vi "Renishaw-XL80_CancelPreHeat.vi"(8 "error in (no error)":errorcluster, 11 "Renishaw-XL80 in":refnum<class "Renishaw-XL80.lvclass">) -> (0 "error out":errorcluster, 3 "Renishaw-XL80 out":refnum<class "Renishaw-XL80.lvclass">)   [LabVIEW 2024, in "Renishaw-XL80.lvclass"]
doc: "This method will terminate the preheat cycle of the ML10. This method should be used with caution, since shortening the preheat cycle may lead to loss of laser stability later.\n\nDefinition\nHRESULTCancelPreheat();\nParameters\nNone\n\nComments\nThis method will return with an HRESULT of E_FAIL if the client has not previously connected to a DX10 by calling Connect. The method will also return E_FAIL if the DX10 is not responding or the ML10 is not responding.\n\nIf the method is successful it will return with an HESULT of S_OK.\n\nNote that this method succeeds even if the ML10 was not in a preheat cycle."
uses:
  Renishaw-XL80.lvclass
  Renishaw-XL80.lvclass/Renishaw-XL80.ctl
  D:/A.C.M/Example CSharp_64/bin/Debug/Interop.DX10SDKADAPTORLib.dll
  Example CSharp_64/bin/Debug/Interop.DX10SDKADAPTORLib.dll
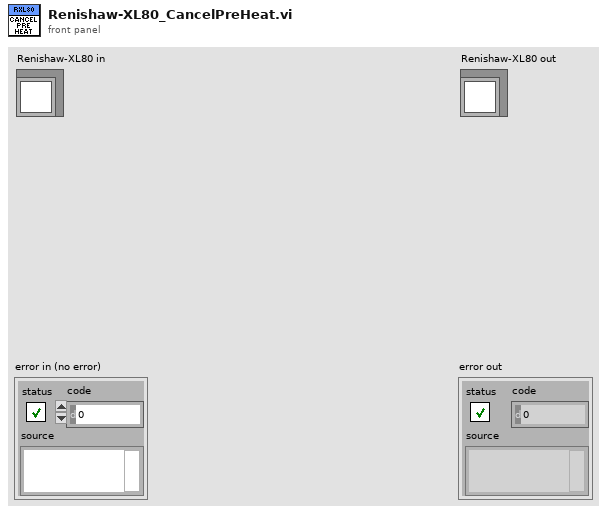
[diagram p1: front panel]
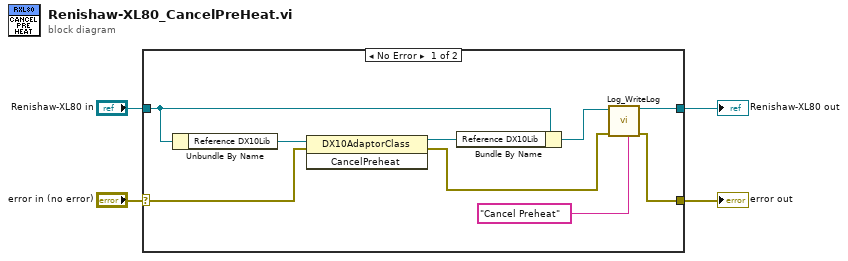
[diagram p0: block diagram]
diagram:
  n1 = case shown="No Error" "error in (no error)" {
    selector: "error in (no error)" -> [w7 w15]
    tunnel: [w5 w15] -> w3
    tunnel: [w8 w14] -> w1
    tunnel: "Renishaw-XL80 in" -> [w9 w14]
    frame No Error {
      n2 = Unbundle By Name(w9) -> ("Reference DX10Lib"=w13:refnum<k24>)
      n3 = invoke class="DX10AdaptorClass" method="CancelPreheat"(reference=w13, error in=w7) -> (reference out=w12:refnum<k24>, error out=w6:errorcluster)  [unwired: 1 in, 1 out]
      n4 = Bundle By Name(cluster=w9, "Reference DX10Lib"=w12) -> (w11:refnum<class "Renishaw-XL80.lvclass">)
      n5 = call-dynamic "Log_WriteLog.vi"("Additional text"="Cancel Preheat", "error in (no error)"=w6, "Log in"=w11) -> ("error out"=w5:errorcluster, "Log out"=w8:refnum<class "Renishaw-XL80.lvclass">)  [unwired: 7 in]
    }
    frame Error {
    }
  }
  "error out" <- w3
  "Renishaw-XL80 out" <- w1
